vi "test-trapezoid-profile-timing-to-negative-goal.vi"() -> ()   [LabVIEW 2019]
uses:
  <vilib>/Rock Robotics/WPI/ThirdParty/JAS_Junk/TrajLib/TRAPEZOID_PROFILE_STATE.ctl
  <vilib>/Rock Robotics/WPI/ThirdParty/JAS_Junk/TrajLib/TRAPEZOID_PROFILE.ctl
  <vilib>/Rock Robotics/WPI/ThirdParty/JAS_Junk/TrajLib/TRAPEZOID_PROFILE_CONSTRAINT.ctl
  <vilib>/Rock Robotics/WPI/ThirdParty/JAS_Junk/TrajLib/TrapProfile_Direct.vi
  <vilib>/Rock Robotics/WPI/ThirdParty/JAS_Junk/TrajLib/TrapProfile_ShouldFlipAcceleration.vi
  <vilib>/Rock Robotics/WPI/ThirdParty/JAS_Junk/TrajLib/Trajectory_Library.lvlib
panel:
  out "ActualTime":dbl
  out "PredictedTImeLeft":dbl
  out "TimeLeftGoal":dbl
  out "TimeLeftPos":dbl
  out "ReachedGoal":bool
  out "TotalTime":dbl
  out "TRAPEZOID_PROFILE":T1 {"Goal"."Velocity" format="%16_6e"; "Goal"."Position" format="%16_6e"; "Initial"."Velocity" format="%16_6e"; "Initial"."Position" format="%16_6e"; "Constraints"."MaxAcceleration" format="%16_6e"; "Constraints"."MaxVelocity" format="%16_6e"; "EndDecel" format="%16_6e"; "EndFullSpeed" format="%16_6e"; "EndAccel" format="%16_6e"}
  out "State":T3 {"Velocity" format="%16_6e"; "Position" format="%16_6e"}
  out "Waveform Chart":T4(graph)
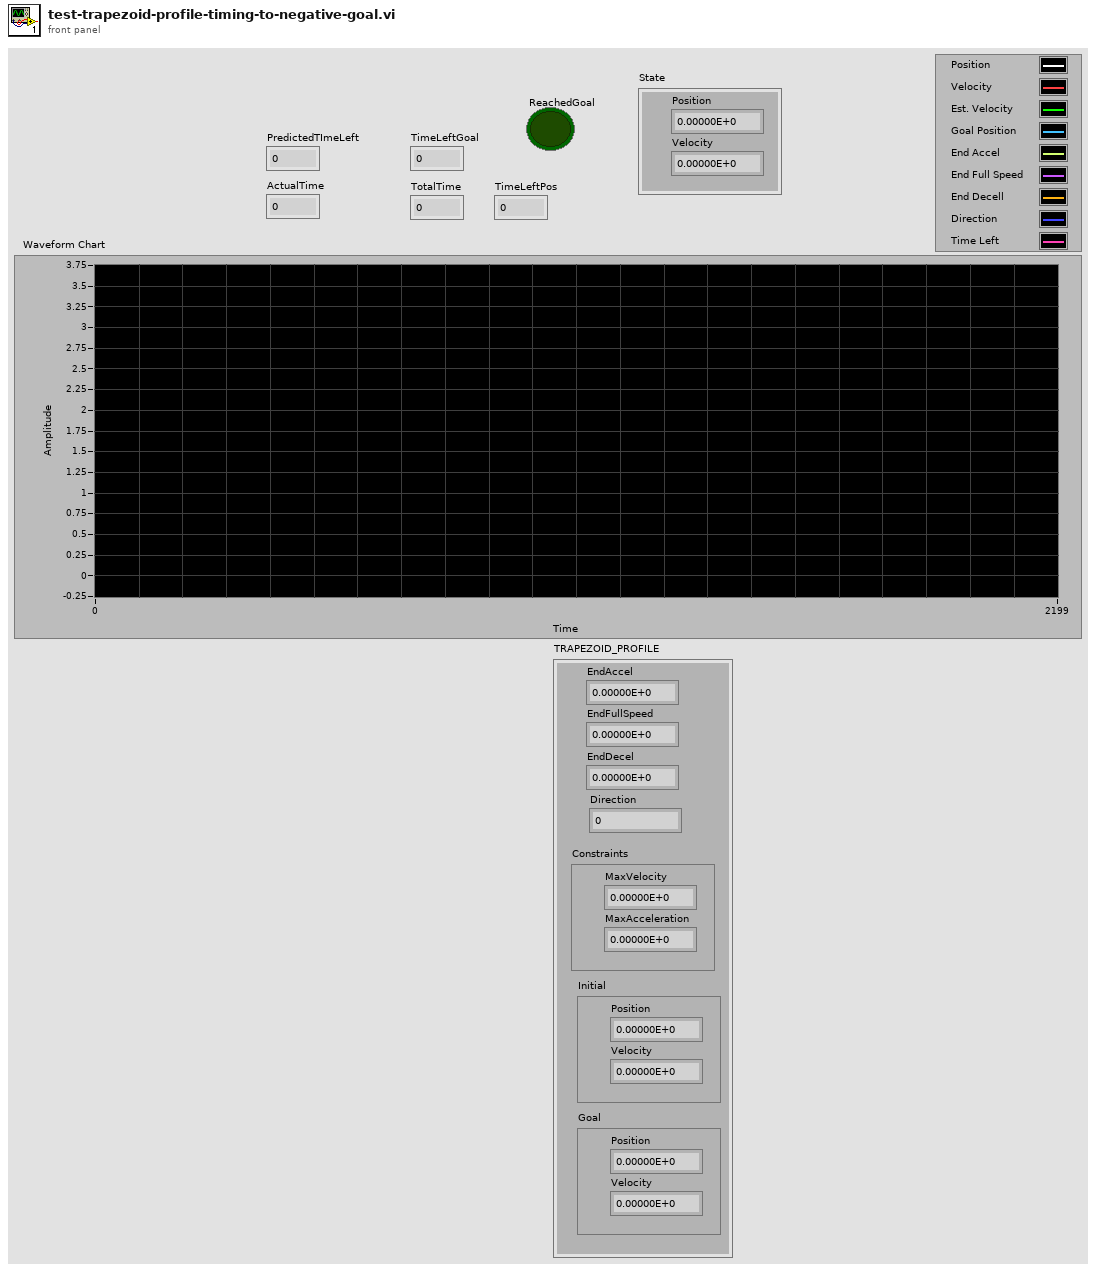
[diagram p1: front panel]
types:
  T1 = typedef "Trajectory_Library.lvlib/TRAPEZOID_PROFILE.ctl" = cluster{"EndAccel":dbl, "EndFullSpeed":dbl, "EndDecel":dbl, "Direction":i32, "Constraints":T2, "Initial":T3, "Goal":T3}
  T2 = typedef "Trajectory_Library.lvlib/TRAPEZOID_PROFILE_CONSTRAINT.ctl" = cluster{"MaxVelocity":dbl, "MaxAcceleration":dbl}
  T3 = typedef "Trajectory_Library.lvlib/TRAPEZOID_PROFILE_STATE.ctl" = cluster{"Position":dbl, "Velocity":dbl}
  T4 = cluster{"Position":dbl, "Velocity":dbl, dbl, "Position":dbl, "EndAccel":dbl, "EndFullSpeed":dbl, "EndDecel":dbl, "Direction":i32, "Position":dbl}
  T5 = cluster{"Position":dbl, "Velocity":dbl, dbl, "Position":dbl, "EndAccel":dbl, "EndFullSpeed":dbl, "EndDecel":dbl, "Direction":i32, "TimeLeft":dbl}
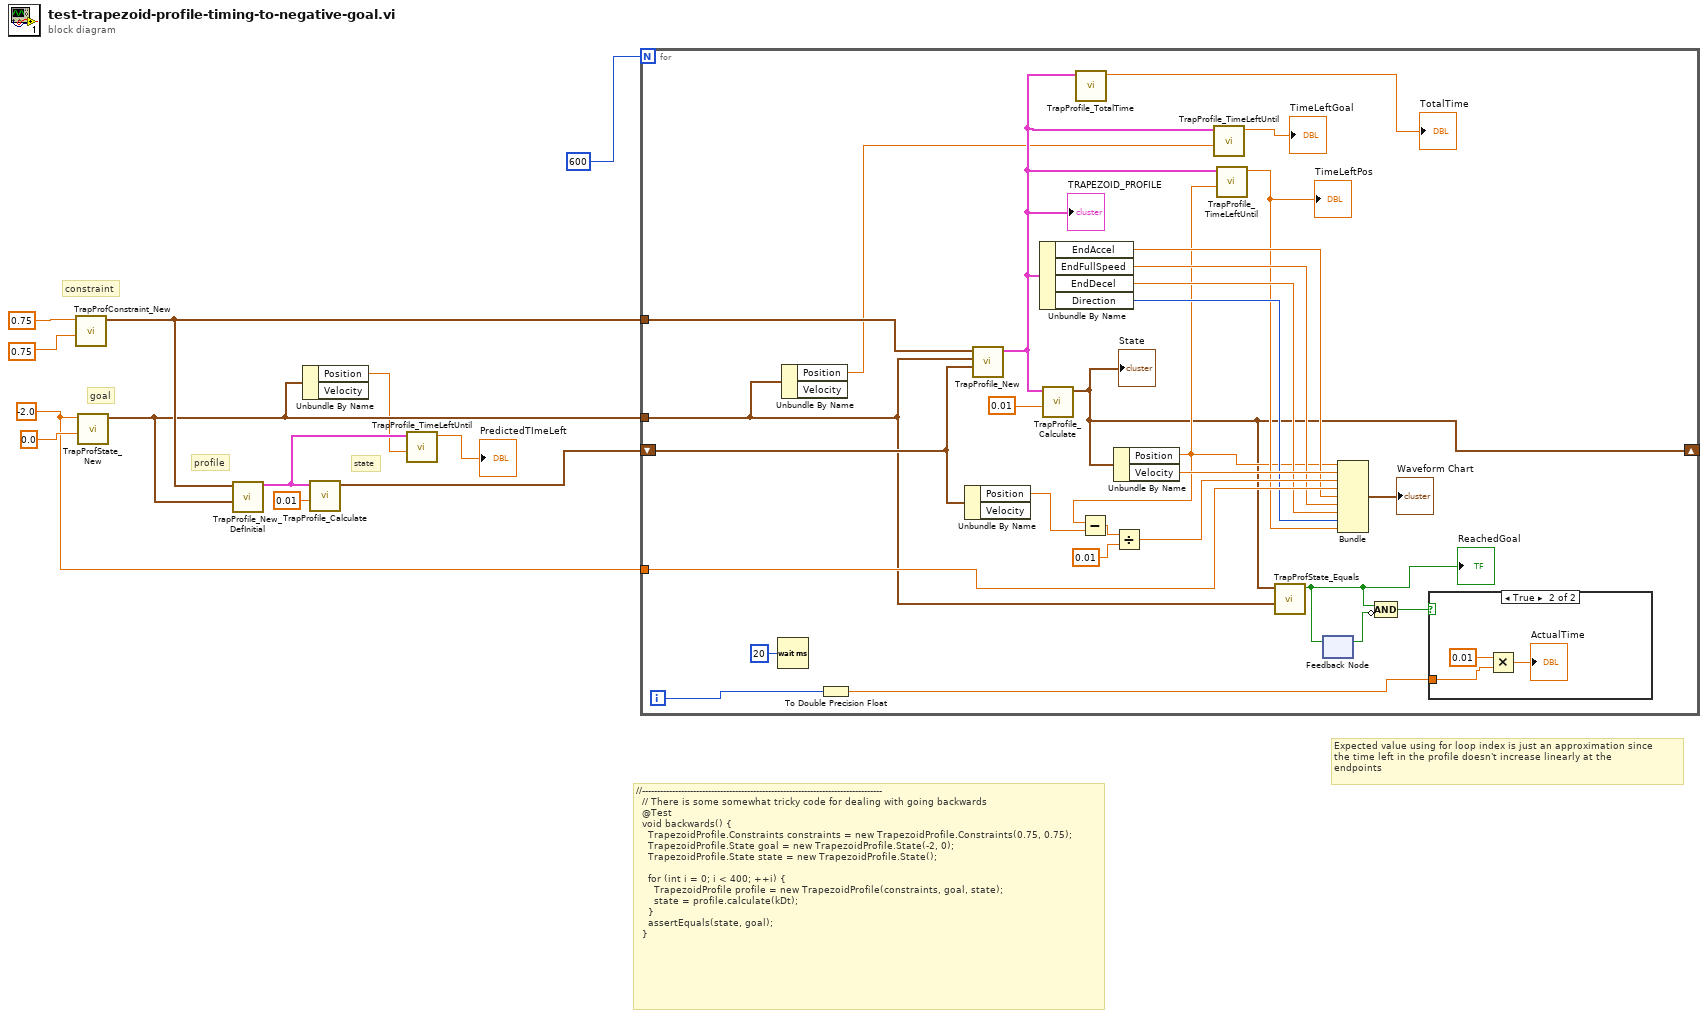
[diagram p0: block diagram]
diagram:
  w8 = -2.0 ("Position")
  # "Expected value using for loop index is just an approximation since\nthe time left in the profile doesn't increase linearly at the\nendpoints"
  # "profile"
  # "state"
  # "//--------------------------------------------------------------------------------\n  // There is some somewhat tricky code for dealing with going backwards\n  @Test\n  void backwards() {\n    TrapezoidProfile.Constraints constraints = new TrapezoidProfile.Constraints(0.75, 0.75);\n    TrapezoidProfile.State goal = new TrapezoidProfile.State(-2, 0);\n    TrapezoidProfile.State state = new TrapezoidProfile.State();\n\n    for (int i = 0; i < 400; ++i) {\n      TrapezoidProfile profile = new TrapezoidProfile(constraints, goal, state);\n      state = profile.calculate(kDt);\n    }\n    assertEquals(state, goal);\n  }"
  # "goal"
  # "constraint"
  n1 = call <vilib>:"TrapProfConstraint_New.vi"("Max Accel"=0.75, "Max Speed (M/S)"=0.75) -> ("TRAPEZOID_PROFILE_CONSTRAINT"=w7:T2)  [unwired: 9 in]
  n2 = call <vilib>:"TrapProfState_New.vi"("Velocity"=0.0, "Position"=w8) -> ("TRAPEZOID_PROFILE_STATE"=w4:T3)  [unwired: 9 in]
  n3 = call <vilib>:"TrapProfile_New_DefInitial.vi"("Goal"=w4, "Constraints"=w7) -> ("TRAPEZOID_PROFILE"=w3:T1)  [unwired: 9 in]
  n4 = Unbundle By Name(w4) -> ("Position"=w2:dbl)  [unwired: 1 out]
  n5 = call <vilib>:"TrapProfile_Calculate.vi"("Time"=0.01, "TRAPEZOID_PROFILE"=w3) -> ("State"=w5:T3)  [unwired: 9 in]
  n6 = call <vilib>:"TrapProfile_TimeLeftUntil.vi"("TargetDistance"=w2, "TRAPEZOID_PROFILE"=w3) -> ("TimeLeft"=→"PredictedTImeLeft":dbl)  [unwired: 9 in]
  n7 = for {
    N: 600 -> [_]
    shift-right: [w22] -> _
    shift-left: w5 -> [w36]
    tunnel: w4 -> [w19]
    tunnel: w8 -> [w32]
    tunnel: w7 -> [w26]
    i -> [w14]
    n8 = Wait (ms)(milliseconds to wait=u32 20) -> ()  [unwired: 1 out]
    n9 = Unbundle By Name(w19) -> ("Position"=w18:dbl)  [unwired: 1 out]
    n10 = To Double Precision Float(number=w14) -> (double precision float=w13:dbl)
    n11 = Unbundle By Name(w36) -> ("Position"=w27:dbl)  [unwired: 1 out]
    n12 = call <vilib>:"TrapProfile_New.vi"("Initial"=w36, "Goal"=w19, "Constraints"=w26) -> ("TRAPEZOID_PROFILE"=w21:T1)  [unwired: 8 in]
    "TRAPEZOID_PROFILE" <- w21
    n13 = Unbundle By Name(w21) -> ("EndAccel"=w31:dbl, "EndFullSpeed"=w30:dbl, "EndDecel"=w29:dbl, "Direction"=w28:i32)
    n14 = call <vilib>:"TrapProfile_Calculate.vi"("Time"=0.01, "TRAPEZOID_PROFILE"=w21) -> ("State"=w22:T3)  [unwired: 9 in]
    "State" <- w22
    n15 = call <vilib>:"TrapProfile_TotalTime.vi"("TRAPEZOID_PROFILE"=w21) -> ("TotalTime"=→"TotalTime":dbl)  [unwired: 10 in]
    n16 = Unbundle By Name(w22) -> ("Position"=w24:dbl, "Velocity"=w38:dbl)
    n17 = Subtract(x=w24, y=w27) -> (x-y=w35:dbl)
    n18 = Divide(x=w35, y=0.01) -> (x/y=w33:dbl)
    n19 = call <vilib>:"TrapProfile_TimeLeftUntil.vi"("TargetDistance"=w18, "TRAPEZOID_PROFILE"=w21) -> ("TimeLeft"=→"TimeLeftGoal":dbl)  [unwired: 9 in]
    n20 = call <vilib>:"TrapProfile_TimeLeftUntil.vi"("TargetDistance"=w24, "TRAPEZOID_PROFILE"=w21) -> ("TimeLeft"=w25:dbl)  [unwired: 9 in]
    "TimeLeftPos" <- w25
    n21 = call <vilib>:"TrapProfState_Equals.vi"("TRAPEZOID_PROFILE_STATE 2"=w19, "TRAPEZOID_PROFILE_STATE"=w22) -> ("Equal"=w17:bool)  [unwired: 9 in]
    "ReachedGoal" <- w17
    n22 = feedback-in #1(w17) -> ()
    n23 = feedback #1() -> (w16:bool)  [unwired: 1 in]
    n24 = Bundle("Position"=w24, "Velocity"=w38, w33, "Position"=w32, "EndAccel"=w31, "EndFullSpeed"=w30, "EndDecel"=w29, "Direction"=w28, "TimeLeft"=w25) -> (→"Waveform Chart":T5)  [unwired: 1 in]
    n25 = Compound Arithmetic op=AND(w17, invert w16) -> (w15:bool)
    n26 = case shown="True" w15 {
      tunnel: w13 -> [_ w43]
      frame False {
      }
      frame True {
        n27 = Multiply(x=0.01, y=w43) -> (x*y=→"ActualTime":dbl)
      }
    }
  }
